vi "Convert From JSON Comp Format.vi"(8 "error in (no error)":errorcluster, 11 "input settings JSON":T1={"sample rate"=51200.0, "range"=5.0, "terminal configuration"=""}) -> (0 "error out":errorcluster, 3 "input settings":T2={"sample rate"=51200.0, "range"=5.0, "terminal configuration"=enum."Pseudodifferential"})   [LabVIEW 2022 SP3, in "Analog Input Settings.lvlib"]
uses:
  Analog Input Settings.lvlib
  service/generation/controls/analog input settings.ctl
  service/generation/controls/terminal configuration.ctl
  analog input settings_json.ctl
  service/generation/controls/AudioGenTypeDefs.lvlib
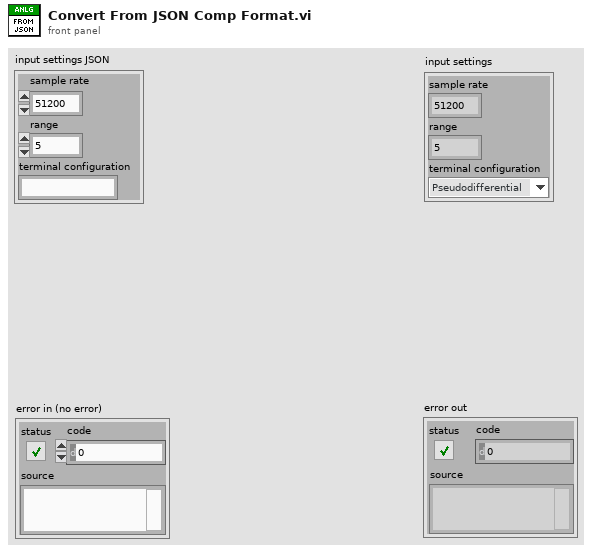
[diagram p1: front panel]
types:
  T1 = typedef "Analog Input Settings.lvlib/analog input settings_json.ctl" = cluster{"sample rate":dbl, "range":dbl, "terminal configuration":string}
  T2 = typedef "AudioGenTypeDefs.lvlib/analog input settings.ctl" = cluster{"sample rate":dbl, "range":dbl, "terminal configuration":T3}
  T3 = typedef "AudioGenTypeDefs.lvlib/terminal configuration.ctl" = enum32{"Default", "RSE", "Differential", "Pseudodifferential"}
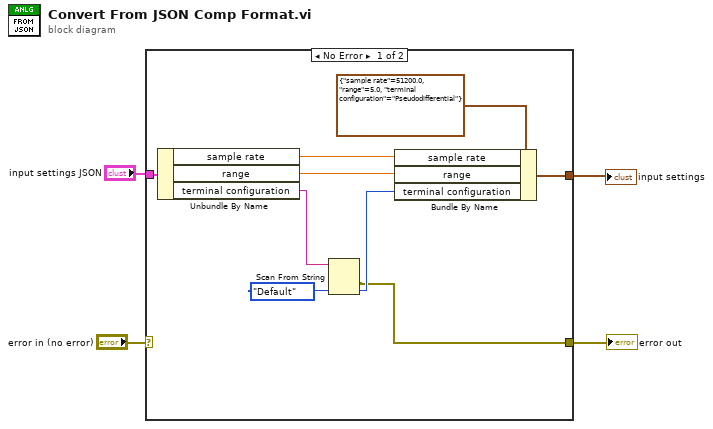
[diagram p0: block diagram]
diagram:
  n1 = case shown="No Error" "error in (no error)" {
    selector: "error in (no error)" -> [_ w14]
    tunnel: [w10 _] -> w4
    tunnel: "input settings JSON" -> [w9 _]
    tunnel: [w5 w14] -> w1
    frame No Error {
      n2 = Unbundle By Name(w9) -> ("sample rate"=w13:dbl, "range"=w12:dbl, "terminal configuration"=w8:string)
      n3 = Scan From String(input string=w8, default 1=terminal_configuration."Default" ("terminal configuration")) -> (error out=w5:errorcluster, output 1=w6:T3)  [unwired: 3 in, 2 out]
      n4 = Bundle By Name(cluster=T2 {"sample rate"=51200.0, "range"=5.0, "terminal configuration"=enum."Pseudodifferential"} ("output settings"), "sample rate"=w13, "range"=w12, "terminal configuration"=w6) -> (w10:T2)
    }
    frame Error {
    }
  }
  "input settings" <- w4
  "error out" <- w1
